vi "SlowButton's.vi"(8 "Speed":dbl, 10 "Straight":bool, 11 "Run":bool) -> ()   [LabVIEW 2018]
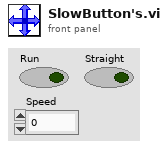
[diagram p1: front panel]
types:
  T1 = typedef "WPI_MotorControlDeviceRef.ctl" = cluster{"DeviceStatus":errorcluster, "Type":T2, "PWM":cluster{"PWM Channel":T3, "DeadBand":T4}, "CAN":cluster{"Device Number":u8, "SetOutput VI Ref":variant, "GetOutput VI Ref":variant, "Enable VI Ref":variant, "Disable VI Ref":variant, "Data":variant}, "Invert":bool, "DIO PWM":cluster{"PWM \"Enable\" Channel":T3, "DIOChannel":T5, "PWM Rate":dbl}}
  T2 = typedef "WPI_MotorControlType.ctl" = enum16{"PWM", "CAN", "DIO PWM"}
  T3 = typedef "FPGA_DIOPWMChannel.ctl" = enum8{"PWM 0", "PWM 1", "PWM 2", "PWM 3", "PWM 4", "PWM 5", "PWM 6", "PWM 7", "PWM 8", "PWM 9", "PWM MXP 0", "PWM MXP 1", "PWM MXP 2", "PWM MXP 3", "PWM MXP 4", "PWM MXP 5", "PWM MXP 6", "PWM MXP 7", "PWM MXP 8", "PWM MXP 9", "Invalid"}
  T4 = typedef "WPI_PWMDeadband.ctl" = cluster{"Name":string, "maxPositivePwm":i32, "minPositivePwm":i32, "centerPwm":i32, "maxNegativePwm":i32, "minNegativePwm":i32, "angularRange":u16}
  T5 = typedef "FPGA_DIOChannel.ctl" = enum8{"DIO 0", "DIO 1", "DIO 2", "DIO 3", "DIO 4", "DIO 5", "DIO 6", "DIO 7", "DIO 8", "DIO 9", "DIO MXP 0", "DIO MXP 1", "DIO MXP 2", "DIO MXP 3", "DIO MXP 4", "DIO MXP 5", "DIO MXP 6", "DIO MXP 7", "DIO MXP 8", "DIO MXP 9", "DIO MXP 10", "DIO MXP 11", "DIO MXP 12", "DIO MXP 13", "DIO MXP 14", "DIO MXP 15", "SPI Port CS1", "SPI Port CS2", "SPI Port CS3", "SPI Port MISO", "SPI Port MOSI", "Invalid"}
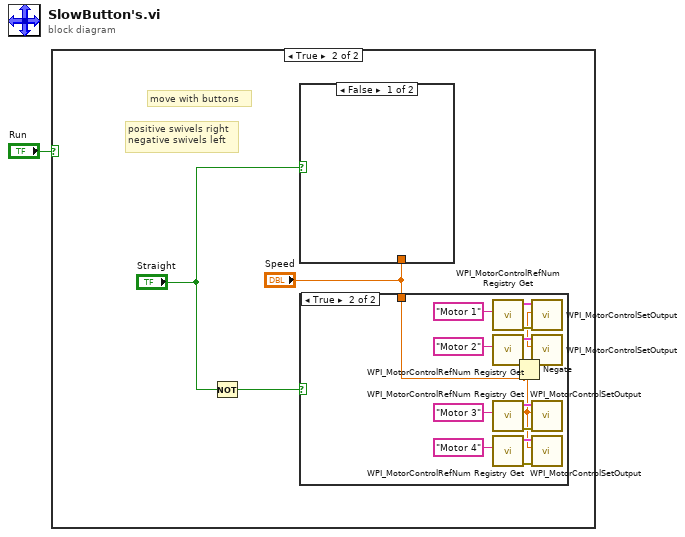
[diagram p0: block diagram]
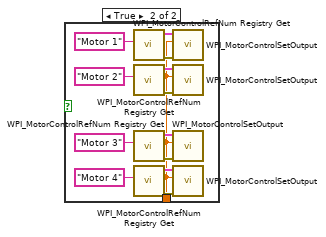
[diagram p4: hidden frame]
diagram:
  n1 = case shown="True" "Run" {
    frame False {
    }
    frame True {
      # "positive swivels right\nnegative swivels left"
      # "move with buttons"
      n2 = Not(x="Straight") -> (.not. x?=w2:bool)
      n3 = case shown="False" "Straight" {
        tunnel: "Speed" -> [_ w19]
        frame False {
        }
        frame True {
          n4 = call <vilib>:"WPI_MotorControlRefNum Registry Get.vi"("refnum name"="Motor 1") -> ("error out"=w30:errorcluster, "MotorControlDevRef"=w31:T1)  [unwired: 9 in]
          n5 = call <vilib>:"WPI_MotorControlRefNum Registry Get.vi"("refnum name"="Motor 2") -> ("error out"=w27:errorcluster, "MotorControlDevRef"=w28:T1)  [unwired: 9 in]
          n6 = call <vilib>:"WPI_MotorControlRefNum Registry Get.vi"("refnum name"="Motor 3") -> ("error out"=w24:errorcluster, "MotorControlDevRef"=w25:T1)  [unwired: 9 in]
          n7 = call <vilib>:"WPI_MotorControlRefNum Registry Get.vi"("refnum name"="Motor 4") -> ("error out"=w21:errorcluster, "MotorControlDevRef"=w22:T1)  [unwired: 9 in]
          n8 = call <vilib>:"WPI_MotorControlSetOutput.vi"("error in (no error)"=w30, "Output"=w19, "MotorControlDevRef"=w31) -> ()  [unwired: 6 in, 3 out]
          n9 = call <vilib>:"WPI_MotorControlSetOutput.vi"("error in (no error)"=w27, "Output"=w19, "MotorControlDevRef"=w28) -> ()  [unwired: 6 in, 3 out]
          n10 = call <vilib>:"WPI_MotorControlSetOutput.vi"("error in (no error)"=w24, "Output"=w19, "MotorControlDevRef"=w25) -> ()  [unwired: 6 in, 3 out]
          n11 = call <vilib>:"WPI_MotorControlSetOutput.vi"("error in (no error)"=w21, "Output"=w19, "MotorControlDevRef"=w22) -> ()  [unwired: 6 in, 3 out]
        }
      }
      n12 = case shown="True" w2 {
        tunnel: "Speed" -> [_ w6]
        frame False {
        }
        frame True {
          n13 = call <vilib>:"WPI_MotorControlRefNum Registry Get.vi"("refnum name"="Motor 1") -> ("error out"=w17:errorcluster, "MotorControlDevRef"=w18:T1)  [unwired: 9 in]
          n14 = call <vilib>:"WPI_MotorControlRefNum Registry Get.vi"("refnum name"="Motor 2") -> ("error out"=w14:errorcluster, "MotorControlDevRef"=w15:T1)  [unwired: 9 in]
          n15 = call <vilib>:"WPI_MotorControlRefNum Registry Get.vi"("refnum name"="Motor 3") -> ("error out"=w11:errorcluster, "MotorControlDevRef"=w12:T1)  [unwired: 9 in]
          n16 = call <vilib>:"WPI_MotorControlRefNum Registry Get.vi"("refnum name"="Motor 4") -> ("error out"=w8:errorcluster, "MotorControlDevRef"=w9:T1)  [unwired: 9 in]
          n17 = Negate(x=w6) -> (-x=w5:dbl)
          n18 = call <vilib>:"WPI_MotorControlSetOutput.vi"("error in (no error)"=w17, "Output"=w5, "MotorControlDevRef"=w18) -> ()  [unwired: 6 in, 3 out]
          n19 = call <vilib>:"WPI_MotorControlSetOutput.vi"("error in (no error)"=w14, "Output"=w5, "MotorControlDevRef"=w15) -> ()  [unwired: 6 in, 3 out]
          n20 = call <vilib>:"WPI_MotorControlSetOutput.vi"("error in (no error)"=w11, "Output"=w6, "MotorControlDevRef"=w12) -> ()  [unwired: 6 in, 3 out]
          n21 = call <vilib>:"WPI_MotorControlSetOutput.vi"("error in (no error)"=w8, "Output"=w6, "MotorControlDevRef"=w9) -> ()  [unwired: 6 in, 3 out]
        }
      }
    }
  }
